vi "Set Logging Root.vi"(8 "error in (no error)":errorcluster, 10 "Logging Root":path, 11 "LoggingManager in":refnum<class "LoggingManager.lvclass">) -> (0 "error out":errorcluster, 3 "LoggingManager out":refnum<class "LoggingManager.lvclass">)   [LabVIEW 2020, in "VolatusData.lvlib" / "LoggingManager.lvclass"]
uses:
  LoggingManager.lvclass
  LoggingManager.lvclass/LoggingManager.ctl
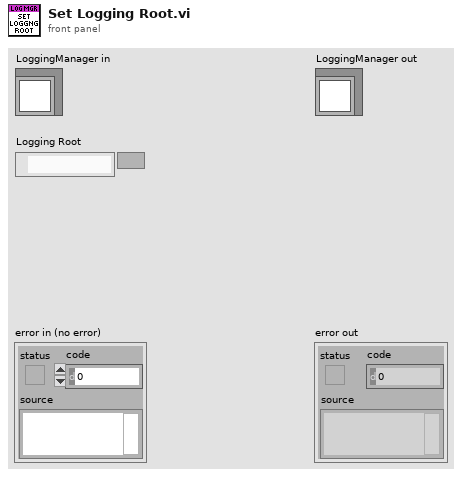
[diagram p1: front panel]
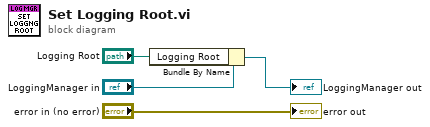
[diagram p0: block diagram]
diagram:
  n1 = Bundle By Name(cluster="LoggingManager in", "Logging Root"="Logging Root") -> (→"LoggingManager out":refnum<class "LoggingManager.lvclass">)
  "error out" <- "error in (no error)"
